vi "F Dwf Digital In Acquisition Mode Get.vi"(8 "error in (no error)":errorcluster, 10 "pacqmode":i32, 11 "hdwf":i32) -> (0 "error out":errorcluster, 2 "pacqmode out":i32, 3 "function return":i32)   [LabVIEW 2019, in "Olasdwf.lvlib"]
doc: "DWFAPI int FDwfDigitalInAcquisitionModeGet(HDWF hdwf, ACQMODE *pacqmode);"
uses:
  Olasdwf.lvlib
  Windows/System32/dwf.dll
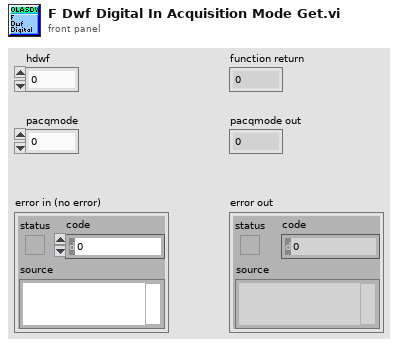
[diagram p1: front panel]
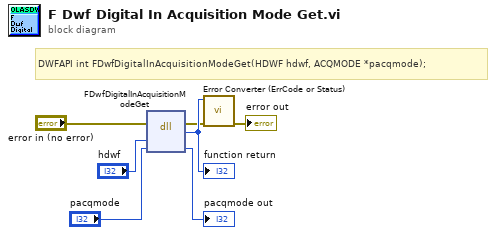
[diagram p0: block diagram]
diagram:
  # "DWFAPI int FDwfDigitalInAcquisitionModeGet(HDWF hdwf, ACQMODE *pacqmode);"
  n1 = dll-call lib="C:/Windows/System32/dwf.*" fn="FDwfDigitalInAcquisitionModeGet"(error in="error in (no error)", "hdwf"="hdwf", "pacqmode"="pacqmode") -> (error out=w2:errorcluster, w7:i32, "pacqmode"=→"pacqmode out":i32)  [unwired: 3 in, 1 out]
  "function return" <- w7
  n2 = call "Error Converter (ErrCode or Status).vi"("error in (no error)"=w2, "error code"=w7) -> ("error out"=→"error out":errorcluster)  [unwired: 9 in]
